vi "Read Key Tap Position.vi"   [LabVIEW 2011, in "LMH-Leap.lvlib"]
doc: "Read key tap gesture positions. Use the polymorphic instance to select between one and N key tap gestures."
uses:
  LMH-Leap.lvlib
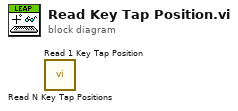
[diagram p0: block diagram]
diagram:
  n1 = call "Read N Key Tap Positions.vi"() -> ()  [unwired: 8 in, 4 out]
  n2 = call "Read 1 Key Tap Position.vi"() -> ()  [unwired: 8 in, 4 out]
